vi "Pkt - Update Packet Order.vi"(8 "error in (no error)":errorcluster, 10 "Channel Names":string[](array[string]), 11 "Node Ptr":T1 format="%.0x") -> (0 "error out":errorcluster, 3 "Node Ptr out":T1 format="%.0x")   [LabVIEW 2016, in "UDP-Custom-Device System Explorer.lvlib"]
uses:
  UDP-Custom-Device System Explorer.lvlib
  <vilib>/NI Veristand/Custom Device API/Custom Device Item Ref.ctl
  <vilib>/NI VeriStand/Custom Device API/Custom Device API.lvlib
  Property Accessors/Shared Section Accessors.lvlib
  Property Accessors/Shared Packet Accessors.lvlib
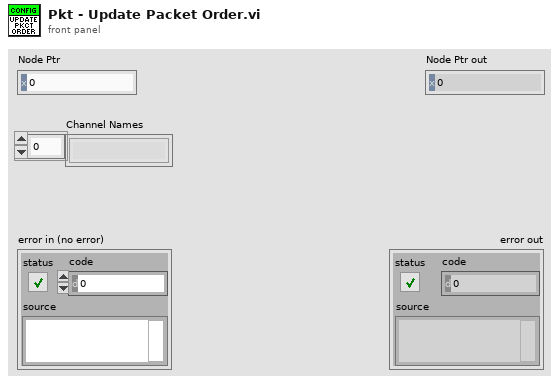
[diagram p1: front panel]
types:
  T1 = typedef "Custom Device API.lvlib/Custom Device Item Ref.ctl" = u64
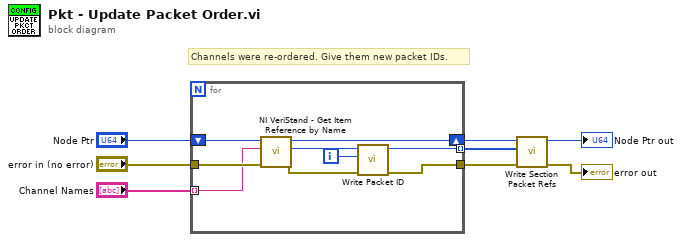
[diagram p0: block diagram]
diagram:
  # "Channels were re-ordered. Give them new packet IDs."
  n1 = for {
    tunnel: "error in (no error)" -> [w17]
    tunnel: "Channel Names" -> [w15] mode=indexing
    shift-right: [w14] -> w5
    shift-left: "Node Ptr" -> [w16]
    tunnel: [w12] -> w1 mode=indexing
    tunnel: [w9] -> w3
    i -> [w11]
    n2 = call <vilib>:"NI VeriStand - Get Item Reference by Name.vi"("error in (no error)"=w17, "Item Name"=w15, "Parent Ref in"=w16) -> ("error out"=w10:errorcluster, "Item Ref"=w13:T1, "Parent Ref out"=w14:T1)  [unwired: 5 in, 1 out]
    n3 = call "Write Packet ID.vi"("error in (no error)"=w10, "Packet ID"=w11, "Node Ptr"=w13) -> ("error out"=w9:errorcluster, "Node Ptr out"=w12:T1)  [unwired: 7 in]
  }
  n4 = call "Write Section Packet Refs.vi"("error in (no error)"=w3, "Dependent Node Refs"=w1, "Node Ptr"=w5) -> ("error out"=→"error out":errorcluster, "Node Ptr out"=→"Node Ptr out":T1)  [unwired: 7 in]
